vi "odor temporal control panel with logging.vi"() -> ()   [LabVIEW 2021]
uses:
  Image Aquisition - Labview/Image Recorder/experiment state global.vi
panel:
  out "flow rates":T1 {"pid reading" format="%0.2f"}
  out "setpoints":T2={"Air "=1.0, "odor1"=0.0, "dilution air"=0.0}
  in  "gradient settings":T3={"background air settings"={"enabled"=FALSE, "temporal ramp type"=enum."Sine", "period(s)"=120.0, "high limit"=100.0, "low limit"=0.0, "duty cycle (sq wave)"=50.0, "phase shift (deg)"=0.0, "value to output when disabled"=0.0}, "odor1 settings"={"enabled"=FALSE, "temporal ramp type"=enum."Sine", "period(s)"=120.0, "high limit"=100.0, "low limit"=0.0, "duty cycle (sq wave)"=50.0, "phase shift (deg)"=0.0, "value to output when disabled"=0.0}, "dilution air"={"enabled"=FALSE, "temporal ramp type"=enum."Sine", "period(s)"=120.0, "high limit"=100.0, "low limit"=0.0, "duty cycle (sq wave)"=50.0, "phase shift (deg)"=0.0, "value to output when disabled"=0.0}} {"dilution air"."value to output when disabled" max=200.0; "dilution air"."low limit" min=0.0 max=200.0 format="%#_6p"; "dilution air"."high limit" max=200.0; "odor1 settings"."value to output when disabled" max=100.0; "odor1 settings"."low limit" min=0.0 max=200.0 format="%#_6p"; "odor1 settings"."high limit" max=100.0; "background air settings"."value to output when disabled" max=5000.0; "background air settings"."low limit" min=0.0 max=50000.0 format="%#_6p"; "background air settings"."high limit" max=5000.0}
  in  "Sync Gradient To Image Aquisition":bool=TRUE
  in  "enable gradient":bool
  in  "restart gradient":bool
  in  "update period (ms)":u32=100
  in  "stop":bool
  out "error out":errorcluster
  # "restarting gradient also enables output"
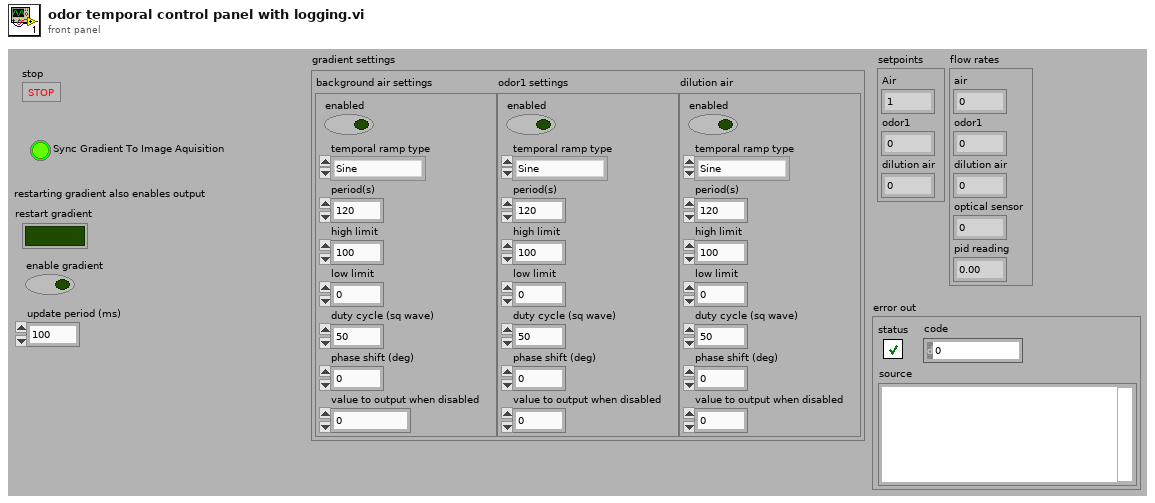
[diagram p1: front panel]
types:
  T1 = cluster{"air":dbl, "odor1":dbl, "dilution air":dbl, "optical sensor":dbl, "pid reading":dbl}
  T2 = cluster{"Air ":dbl, "odor1":dbl, "dilution air":dbl}
  T3 = cluster{"background air settings":cluster{"enabled":bool, "temporal ramp type":enum16{"Sine", "Triangle", "Sawtooth", "Square", "Exponential"}, "period(s)":dbl, "high limit":dbl, "low limit":dbl, "duty cycle (sq wave)":dbl, "phase shift (deg)":dbl, "value to output when disabled":dbl}, "odor1 settings":cluster{"enabled":bool, "temporal ramp type":enum16{"Sine", "Triangle", "Sawtooth", "Square", "Exponential"}, "period(s)":dbl, "high limit":dbl, "low limit":dbl, "duty cycle (sq wave)":dbl, "phase shift (deg)":dbl, "value to output when disabled":dbl}, "dilution air":cluster{"enabled":bool, "temporal ramp type":enum16{"Sine", "Triangle", "Sawtooth", "Square", "Exponential"}, "period(s)":dbl, "high limit":dbl, "low limit":dbl, "duty cycle (sq wave)":dbl, "phase shift (deg)":dbl, "value to output when disabled":dbl}}
  T4 = typedef "LabJack AOAI Channel.ctl" = cluster{"handle":i32, "Channel":i32, "IOType":string, "Scaling":dbl}
  T5 = cluster{"Input Labjack Tasks":cluster{"OdorFlowRate":T4, "PID":T4, "Optical Flow Sensor":T4, "Background Air Flow":T4, "Air Dilution":T4}, "Output Labjack Tasks":cluster{"OdorFlowRate":T4, "Background Air Flow":T4, "Air Dilution":T4}}
  T6 = cluster{"experiment started":bool, "experiment ended":bool, "experiment start time":u32}
  T7 = cluster{"Air ":dbl, "odor1":dbl, "diltuon air":dbl}
  T8 = cluster{"data directory":path, "file stub":string}
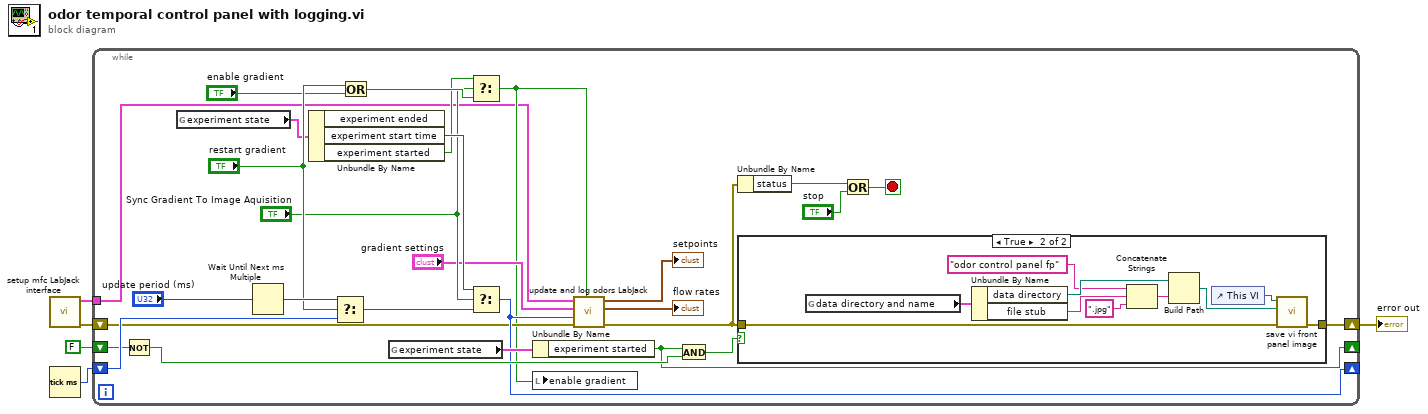
[diagram p0: block diagram]
diagram:
  n1 = call "setup mfc LabJack interface.vi"() -> ("error out"=w4:errorcluster, "LabJack Tasks"=w1:T5)  [unwired: 10 in]
  n2 = Tick Count (ms)() -> (millisecond timer value=w5:u32)
  n3 = while {
    shift-right: [w14] -> w3
    shift-left: w4 -> [w11]
    shift-right: [w12] -> _
    shift-left: w5 -> [w30]
    tunnel: w1 -> [w9]
    shift-right: [w16] -> _
    shift-left: FALSE ("experiment started") -> [w15]
    stop <- w33 stop-if-true
    n4 = Not(x=w15) -> (.not. x?=w19:bool)
    n5 = global read "experiment state global.vi" "experiment state"() -> (w25:T6)
    n6 = Wait Until Next ms Multiple(millisecond multiple="update period (ms)") -> (millisecond timer value=w29:u32)
    n7 = Unbundle By Name(w25) -> ("experiment start time"=w24:u32, "experiment started"=w20:bool)  [unwired: 1 out]
    n8 = Select(t=w29, s="restart gradient", f=w30) -> (s? t:f=w26:u32)
    n9 = Or(x="restart gradient", y="enable gradient") -> (x .or. y?=w23:bool)
    n10 = global read "experiment state global.vi" "experiment state"() -> (w17:T6)
    n11 = Select(t=w20, s="Sync Gradient To Image Aquisition", f=w23) -> (s? t:f=w10:bool)
    n12 = Select(t=w24, s="Sync Gradient To Image Aquisition", f=w26) -> (s? t:f=w12:u32)
    n13 = Unbundle By Name(w17) -> ("experiment started"=w16:bool)
    n14 = local write "enable gradient"(w10) -> ()
    n15 = call "update and log odors LabJack.vi"("global enable"=w10, "error in"=w11, "t0"=w12, "gradient settings"="gradient settings", "LabJack Tasks"=w9) -> ("error out"=w8:errorcluster, "flow rates"=→"flow rates":T1, "setpoints"=→"setpoints":T7)  [unwired: 4 in]
    n16 = And(x=w16, y=w19) -> (x .and. y?=w18:bool)
    n17 = Unbundle By Name(w8) -> ("status"=w27:bool)
    n18 = case shown="True" w18 {
      tunnel: [w34 w36] -> w14
      tunnel: w8 -> [w34 w35]
      frame False {
      }
      frame True {
        n19 = global read "experiment state global.vi" "data directory and name"() -> (w43:T8)
        n20 = Unbundle By Name(w43) -> ("data directory"=w42:path, "file stub"=w41:string)
        n21 = Concatenate Strings("odor control panel fp" ("string"), w41, ".jpg" ("string")) -> (w38:string)
        n22 = Build Path(base path=w42, name or relative path=w38) -> (appended path=w37:path)
        n23 = control-ref of="This VI"() -> (w44:refnum<vi>)
        n24 = call "save vi front panel image.vi"("error in (no error)"=w35, "path to JPEG file"=w37, "This VI"=w44) -> ("error out"=w36:errorcluster)  [unwired: 8 in]
      }
    }
    n25 = Or(x=w27, y="stop") -> (x .or. y?=w33:bool)
  }
  "error out" <- w3
